vi "OpenXL_WorkSheet By Index.vi"(8 "error in (no error)":errorcluster, 10 "Index(1)":i32=1, 11 "Refnum Cluster In":T1) -> (0 "error out":errorcluster, 3 "Refnum Cluster Out":T2)   [LabVIEW 2015]
doc: "This VI opens the specified worksheet for the open workbook. Pair this VI with CloseXL_Worksheet.vi.\n\nThe Sheet input is variant data type, so you can specify the sheet by its title (string) or by its number (1,2,3, etc.)."
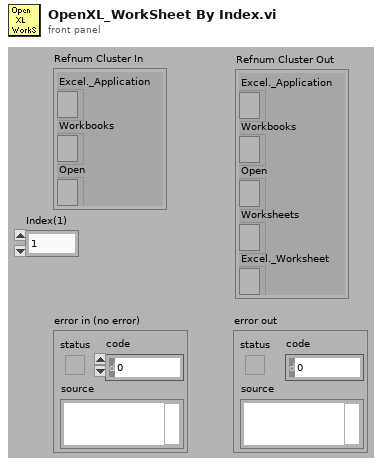
[diagram p1: front panel]
types:
  T1 = cluster{"Excel._Application":refnum<k7>, "Workbooks":refnum<k7>, "Open":refnum<k7>}
  T2 = cluster{"Excel._Application":refnum<k7>, "Workbooks":refnum<k7>, "Open":refnum<k7>, "Worksheets":refnum<k7>, "Excel._Worksheet":refnum<k7>}
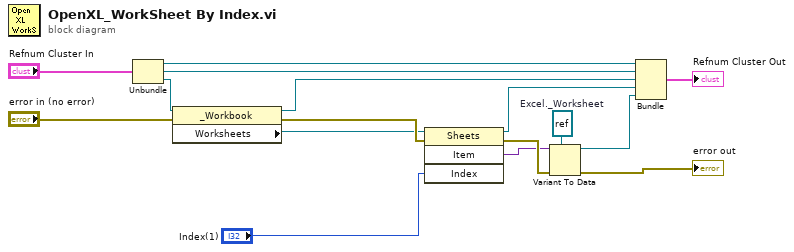
[diagram p0: block diagram]
diagram:
  w11 = refnum<k7> refnum  # Excel._Worksheet
  n1 = Unbundle("Refnum Cluster In") -> ("Excel._Application"=w8:refnum<k7>, "Workbooks"=w9:refnum<k7>, "Open"=w7:refnum<k7>)
  n2 = property class="_Workbook"(reference=w7, error in="error in (no error)") -> (reference out=w15:refnum<k7>, error out=w12:errorcluster, "Worksheets"=w3:refnum<k7>)
  n3 = invoke class="Sheets" method="Item"(reference=w3, error in=w12, "Index"="Index(1)") -> (reference out=w16:refnum<k7>, error out=w13:errorcluster, "Item"=w10:variant)  [unwired: 1 in, 1 out]
  n4 = Variant To Data(error in=w13, type=w11, Variant=w10) -> (data=w2:refnum<k7>, error out=→"error out":errorcluster)
  n5 = Bundle("Excel._Application"=w8, "Workbooks"=w9, "Open"=w15, "Worksheets"=w16, "Excel._Worksheet"=w2) -> (→"Refnum Cluster Out":T2)  [unwired: 1 in]
